vi "RichToFlatw4lvgrpc_Msg_ToClient_4.vi"(5 "OutputClusterType":T1, 11 "InputCluster":T2) -> (3 "OutputCluster":T1)   [LabVIEW 2019, in "Generated_server.lvlib"]
uses:
  Generated_server.lvlib
  w4lvgrpc_Msg_ToClient_4_Flat.ctl
  w4lvgrpc_Msg_ToClient_4.ctl
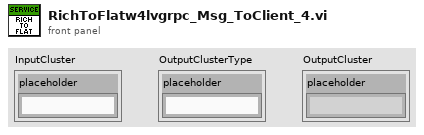
[diagram p1: front panel]
types:
  T1 = typedef "Generated_server.lvlib/w4lvgrpc_Msg_ToClient_4_Flat.ctl" = cluster{"placeholder":string}
  T2 = typedef "Generated_server.lvlib/w4lvgrpc_Msg_ToClient_4.ctl" = cluster{"placeholder":string}
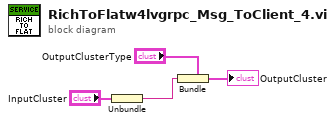
[diagram p0: block diagram]
diagram:
  n1 = Unbundle "Unbundle"("InputCluster") -> ("placeholder"=w1:string)
  n2 = Bundle "Bundle"(cluster="OutputClusterType", "placeholder"=w1) -> (→"OutputCluster":T1)
